vi "ConfigUtilities - Init Rx Packet Page.vi"(7 "Rx Section Cluster In":T2, 8 "error in (no error)":errorcluster, 11 "Node Ptr In":T1 format="%.0x") -> (0 "error out":errorcluster, 3 "Node Ptr Out":T1 format="%.0x", 5 "Rx Section Cluster Out":T2)   [LabVIEW 2016, in "UDP-Custom-Device System Explorer.lvlib"]
uses:
  UDP-Custom-Device System Explorer.lvlib
  Types/TypeDef - Rx Section Page References.ctl
  <vilib>/NI Veristand/Custom Device API/Custom Device Item Ref.ctl
  Shared/Constants.vi
  <vilib>/NI Veristand/Custom Device API/Get Item Property (I32).vi
  <vilib>/NI Veristand/Custom Device API/Get Item Property (Boolean).vi
  <vilib>/NI Veristand/Custom Device API/Get Item Property (String).vi
  <vilib>/NI VeriStand/Custom Device API/Custom Device API.lvlib
  Shared/UDP-Custom-Device Shared.lvlib
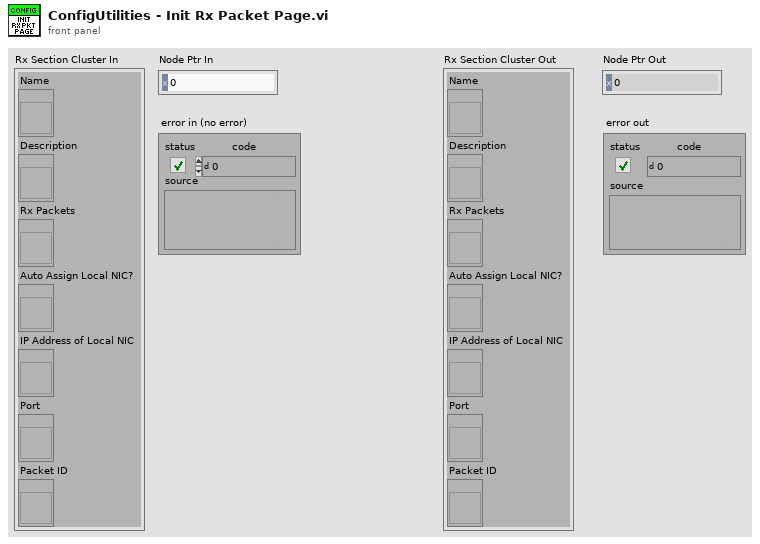
[diagram p1: front panel]
types:
  T1 = typedef "Custom Device API.lvlib/Custom Device Item Ref.ctl" = u64
  T2 = typedef "UDP-Custom-Device System Explorer.lvlib/TypeDef - Rx Section Page References.ctl" = cluster{"Name":refnum<vi>, "Description":refnum<vi>, "Rx Packets":refnum<vi>, "Auto Assign Local NIC?":refnum<vi>, "IP Address of Local NIC":refnum<vi>, "Port":refnum<vi>, "Packet ID":refnum<vi>}
  T3 = typedef "Custom Device API.lvlib/Custom Device Item Info.ctl" = cluster{"Name":string, "Is Channel":bool, "GUID":string, "Is Waveform":bool}
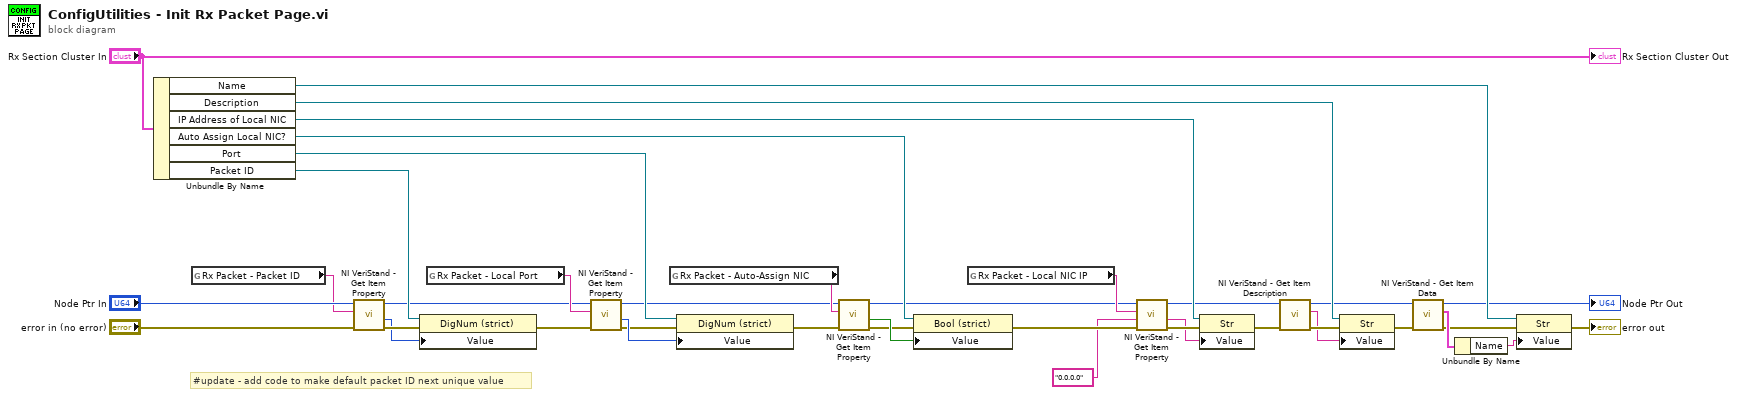
[diagram p0: block diagram]
diagram:
  # "#update - add code to make default packet ID next unique value"
  n1 = Unbundle By Name("Rx Section Cluster In") -> ("Name"=w19:refnum<vi>, "Description"=w18:refnum<vi>, "IP Address of Local NIC"=w4:refnum<vi>, "Auto Assign Local NIC?"=w9:refnum<vi>, "Port"=w24:refnum<vi>, "Packet ID"=w33:refnum<vi>)
  n2 = global read "Constants.vi" "Rx Packet - Packet ID"() -> (w35:string)
  n3 = call-poly <vilib>:"NI VeriStand - Get Item Property.vi"("error in (no error)"="error in (no error)", "Property Name"=w35, "Item Ref in"="Node Ptr In") -> ("error out"=w34:errorcluster, "Value"=w32:i32, "Item Ref out"=w25:T1)  [unwired: 5 in, 1 out]
  n4 = property class="DigNum (strict)"(reference=w33, error in=w34, "Value"=w32) -> (error out=w23:errorcluster)  [unwired: 1 out]
  n5 = global read "Constants.vi" "Rx Packet - Local Port"() -> (w29:string)
  n6 = call-poly <vilib>:"NI VeriStand - Get Item Property.vi"("error in (no error)"=w23, "Property Name"=w29, "Item Ref in"=w25) -> ("error out"=w30:errorcluster, "Value"=w31:i32, "Item Ref out"=w8:T1)  [unwired: 5 in, 1 out]
  n7 = global read "Constants.vi" "Rx Packet - Auto-Assign NIC"() -> (w20:string)
  n8 = property class="DigNum (strict)"(reference=w24, error in=w30, "Value"=w31) -> (error out=w7:errorcluster)  [unwired: 1 out]
  n9 = call-poly <vilib>:"NI VeriStand - Get Item Property.vi"("error in (no error)"=w7, "Property Name"=w20, "Item Ref in"=w8) -> ("error out"=w21:errorcluster, "Value"=w22:bool, "Item Ref out"=w6:T1)  [unwired: 5 in, 1 out]
  n10 = property class="Bool (strict)"(reference=w9, error in=w21, "Value"=w22) -> (error out=w5:errorcluster)  [unwired: 1 out]
  n11 = global read "Constants.vi" "Rx Packet - Local NIC IP"() -> (w28:string)
  n12 = call-poly <vilib>:"NI VeriStand - Get Item Property.vi"("error in (no error)"=w5, "Default Value"="0.0.0.0", "Property Name"=w28, "Item Ref in"=w6) -> ("error out"=w27:errorcluster, "Value"=w26:string, "Item Ref out"=w1:T1)  [unwired: 4 in, 1 out]
  n13 = property class="Str"(reference=w4, error in=w27, "Value"=w26) -> (error out=w2:errorcluster)  [unwired: 1 out]
  n14 = call <vilib>:"NI VeriStand - Get Item Description.vi"("error in (no error)"=w2, "Item Ref in"=w1) -> ("error out"=w17:errorcluster, "Description"=w16:string, "Item Ref out"=w14:T1)  [unwired: 7 out]
  n15 = property class="Str"(reference=w18, error in=w17, "Value"=w16) -> (error out=w15:errorcluster)  [unwired: 1 out]
  n16 = call <vilib>:"NI VeriStand - Get Item Data.vi"("error in (no error)"=w15, "Item Ref in"=w14) -> ("error out"=w38:errorcluster, "Item Info"=w39:T3, "Item Ref out"=→"Node Ptr Out":T1)  [unwired: 6 in, 1 out]
  n17 = Unbundle By Name(w39) -> ("Name"=w13:string)
  n18 = property class="Str"(reference=w19, error in=w38, "Value"=w13) -> (error out=→"error out":errorcluster)  [unwired: 1 out]
  "Rx Section Cluster Out" <- "Rx Section Cluster In"
